vi "_replaceUsiForbiddenCharacters.vi"(4 "error in (no error)":errorcluster, 6 "replace with this char (_)":string="_", 7 "string in":string) -> (0 "error out":errorcluster, 3 "string out":string)   [LabVIEW 2020]
uses:
  usiForbiddenCharacters.ctl
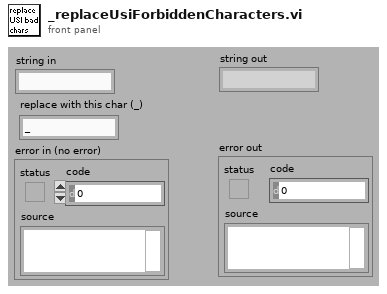
[diagram p1: front panel]
types:
  T1 = typedef "usiForbiddenCharacters.ctl" = string[]
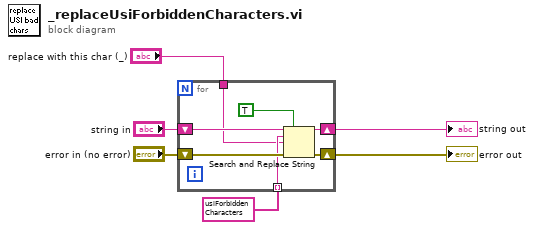
[diagram p0: block diagram]
diagram:
  n1 = for {
    shift-right: [w13] -> w2
    shift-left: "error in (no error)" -> [w11]
    shift-right: [w12] -> w3
    shift-left: "string in" -> [w10]
    tunnel: T1 [".", ":", ",", ";", "'", "\\", "@", "<", ">", "#", "[", "]", "%", "(", ")", "{", "}", "|", "*", "?", "=", "!", "\"", "^", "$", "&", "+", "-", "/", " "] ("USI Forbidden Characters") -> [w9] mode=indexing
    tunnel: "replace with this char (_)" -> [w7]
    n2 = Search and Replace String(replace all?=TRUE ("replace all? (F)"), input string=w10, search string=w9, replace string=w7, error in=w11) -> (result string=w12:string, error out=w13:errorcluster)  [unwired: 3 in, 2 out]
  }
  "string out" <- w3
  "error out" <- w2
